vi "Serial_Init(SubVI).vi"(0 "VISA Refnum in":refnum<visa-resource-name>="COM7", 2 "wbc":dbl=1.0, 3 "delay before read (ms)":u32=265, 4 "baud rate":u32=115200, 7 "data bits":u16=8 min=5 max=8 step=1, 9 "parity":u16(ring) items=["None", "Odd", "Even", "Mark", "Space"], 11 "stop bits":u16(ring)=10 items=["1.0"=10, "1.5"=15, "2.0"=20], 12 "Success":i32, 13 "flow control":u16(ring) items=["None"=0, "XON/XOFF"=1, "RTS/CTS"=2, "DTR/DSR"=4]) -> (10 "Success_out":i32, 14 "VISA out":refnum<visa-resource-name>="COM7", 15 "read string":string, 19 "error out":errorcluster)   [LabVIEW 2017]
uses:
  <vilib>/Instr/_visa.llb/VISA Configure Serial Port (Instr).vi
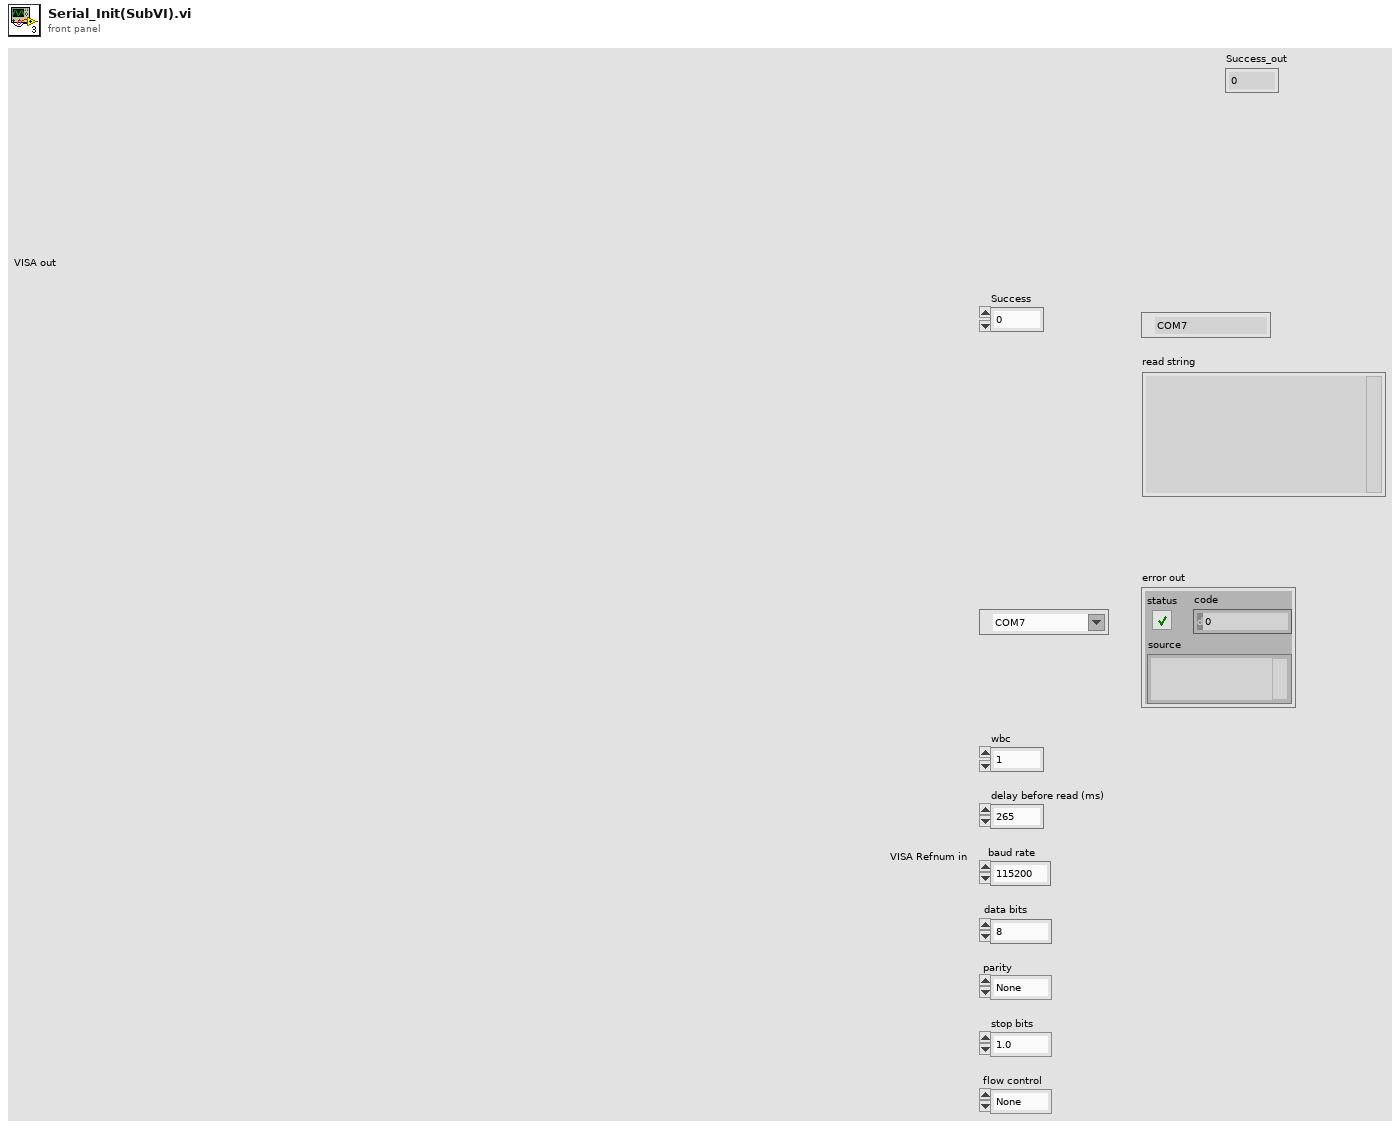
[diagram p1: front panel]
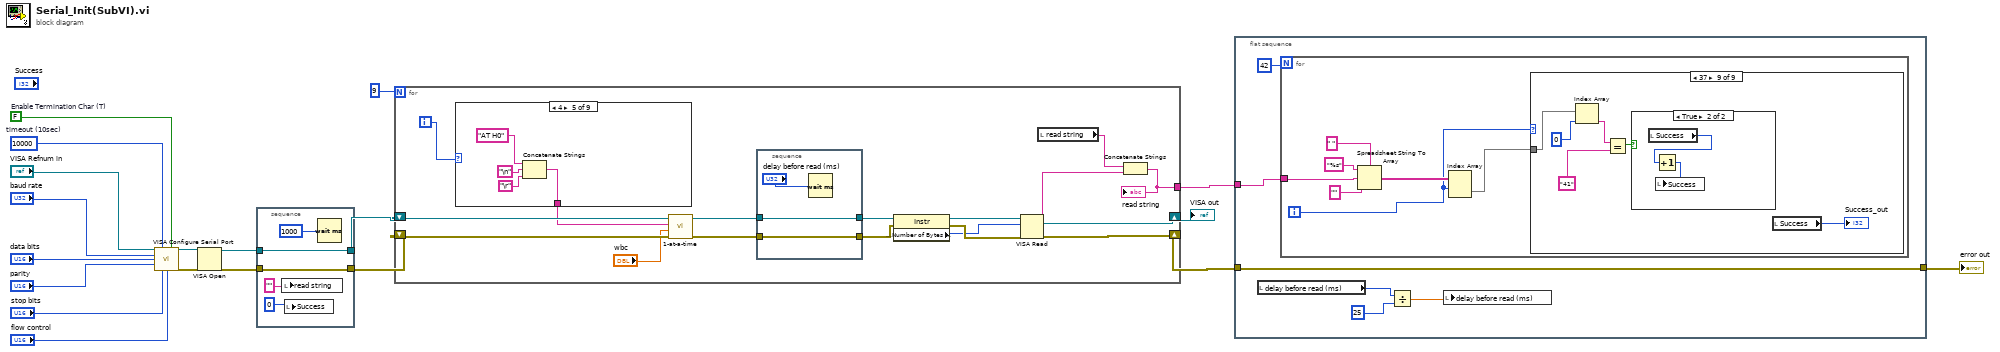
[diagram p0: block diagram]
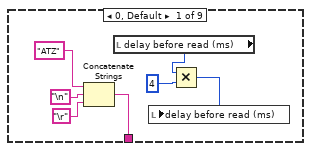
[diagram p2: hidden frame]
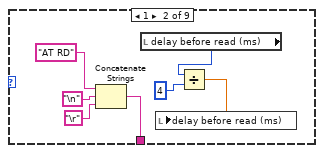
[diagram p3: hidden frame]
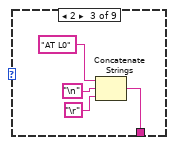
[diagram p4: hidden frame]
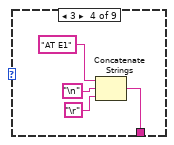
[diagram p5: hidden frame]
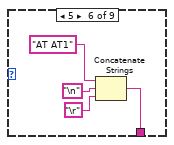
[diagram p6: hidden frame]
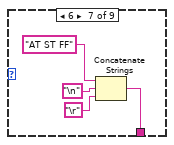
[diagram p7: hidden frame]
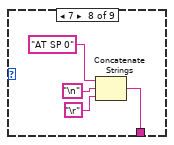
[diagram p8: hidden frame]
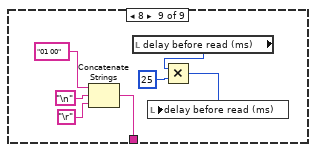
[diagram p9: hidden frame]
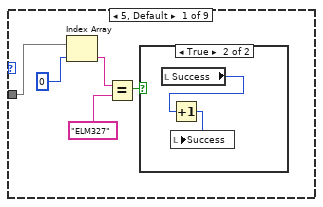
[diagram p10: hidden frame]
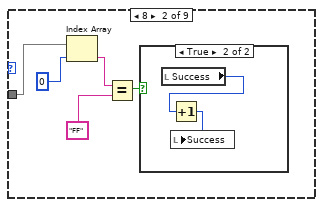
[diagram p12: hidden frame]
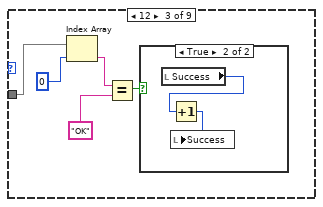
[diagram p14: hidden frame]
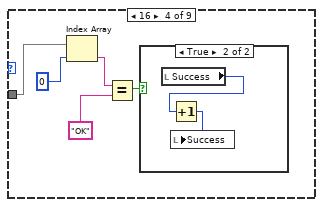
[diagram p16: hidden frame]
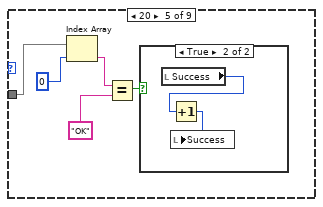
[diagram p18: hidden frame]
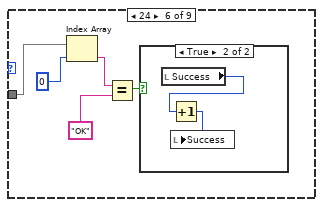
[diagram p20: hidden frame]
diagram:
  w5 = FALSE  # Enable Termination Char (T)
  w4 = u32 10000  # timeout (10sec)
  n1 = call-poly "VISA Configure Serial Port"("VISA resource name"="VISA Refnum in", "timeout (10sec)"=w4, "Enable Termination\nChar (T)"=w5, "baud rate (9600)"="baud rate", "data bits (8)"="data bits", "parity (0:none)"="parity", "stop bits (10: 1 bit)"="stop bits", "flow control (0:none)"="flow control") -> ("VISA resource name out"=w9:refnum<visa-resource-name>, "error out"=w10:errorcluster)  [unwired: 6 in]
  n2 = VISA Open(error in (no error)=w10, VISA resource name=w9) -> (VISA resource name=w11:refnum<visa-resource-name>, error out=w12:errorcluster)  [unwired: 3 in]
  n3 = stacked-sequence {
    tunnel: w12 -> [w24]
    tunnel: [w24] -> w14
    tunnel: w11 -> [w23]
    tunnel: [w23] -> w13
    frame #0 {
      n4 = local write "read string"("") -> ()
      n5 = local write "Success"(0) -> ()
      n6 = Wait (ms)(milliseconds to wait=u32 1000 ("delay before read (ms) 2")) -> ()  [unwired: 1 out]
    }
  }
  n7 = for {
    N: 9 -> [_]
    shift-right: [w29] -> w16
    shift-left: w14 -> [w40]
    shift-right: [w30] -> w15
    shift-left: w13 -> [w41]
    tunnel: [w28] -> w18
    i -> [w26]
    n8 = case shown="4" w26 {
      tunnel: [w48 w55 w59 w63 w67 w71 w75 w79 w86] -> w38
      frame 0, Default {
        n9 = Concatenate Strings("ATZ" ("string to write"), "\n", "\r") -> (w48:string)
        n10 = local read "delay before read (ms)"() -> (w43:u32)
        n11 = Multiply(x=w43, y=4) -> (x*y=w42:u32)
        n12 = local write "delay before read (ms)"(w42) -> ()
      }
      frame 1 {
        n13 = Concatenate Strings("AT RD" ("string to write"), "\n", "\r") -> (w55:string)
        n14 = local read "delay before read (ms)"() -> (w51:u32)
        n15 = Divide(x=w51, y=4) -> (x/y=w49:dbl)
        n16 = local write "delay before read (ms)"(w49) -> ()
      }
      frame 2 {
        n17 = Concatenate Strings("AT L0" ("string to write"), "\n", "\r") -> (w59:string)
      }
      frame 3 {
        n18 = Concatenate Strings("AT E1" ("string to write"), "\n", "\r") -> (w63:string)
      }
      frame 4 {
        n19 = Concatenate Strings("AT H0" ("string to write"), "\n", "\r") -> (w67:string)
      }
      frame 5 {
        n20 = Concatenate Strings("AT AT1" ("string to write"), "\n", "\r") -> (w71:string)
      }
      frame 6 {
        n21 = Concatenate Strings("AT ST FF" ("string to write"), "\n", "\r") -> (w75:string)
      }
      frame 7 {
        n22 = Concatenate Strings("AT SP 0" ("string to write"), "\n", "\r") -> (w79:string)
      }
      frame 8 {
        n23 = Concatenate Strings("01 00" ("string to write"), "\n", "\r") -> (w86:string)
        n24 = local read "delay before read (ms)"() -> (w81:u32)
        n25 = Multiply(x=w81, y=25) -> (x*y=w80:u32)
        n26 = local write "delay before read (ms)"(w80) -> ()
      }
    }
    n27 = call "1-at-a-time.vi"("error in (no error)"=w40, "Wait Between Characters(ms)"="wbc", "write buffer"=w38, "VISA resource name"=w41) -> ("error out"=w36:errorcluster, "VISA resource name out"=w37:refnum<visa-resource-name>)  [unwired: 5 in, 1 out]
    n28 = stacked-sequence {
      tunnel: w36 -> [w89]
      tunnel: [w89] -> w31
      tunnel: w37 -> [w88]
      tunnel: [w88] -> w32
      frame #0 {
        n29 = Wait (ms)(milliseconds to wait="delay before read (ms)") -> ()  [unwired: 1 out]
      }
    }
    n30 = property class="Instr"(reference=w32, error in=w31) -> (reference out=w35:refnum<visa-resource-name>, error out=w34:errorcluster, "Serial Settings:Number of Bytes at Serial Port"=w33:u32)
    n31 = VISA Read(VISA resource name=w35, byte count=w33, error in (no error)=w34) -> (VISA resource name out=w30:refnum<visa-resource-name>, read buffer=w27:string, error out=w29:errorcluster)  [unwired: 1 out]
    n32 = local read "read string"() -> (w25:string)
    n33 = Concatenate Strings(w25, w27) -> (w28:string)
    "read string" <- w28
  }
  "VISA out" <- w15
  n34 = flat-sequence {
    tunnel: w16 -> [w95]
    tunnel: [w95] -> w17
    tunnel: w18 -> [w94]
    frame #0 {
      n35 = local read "delay before read (ms)"() -> (w90:u32)
      n36 = for {
        N: 42 -> [_]
        tunnel: w94 -> [w98]
        i -> [w97]
        n37 = Spreadsheet String To Array(delimiter (Tab)=" ", format string="%s" ("spreadsheet string"), spreadsheet string=w98, array type (2D Dbl)="" ("spreadsheet string")) -> (array=w102:string[][])
        n38 = Index Array(array=w102, index (row)=w97) -> (element=w96:string[])  [unwired: 1 in]
        n39 = case shown="37" w97 {
          tunnel: w96 -> [w107 w114 w121 w128 w135 w142 w149 w156 w164]
          frame 5, Default {
            n40 = Index Array(array=w107, index=0) -> (element=w105:string)
            n41 = Equal?(x=w105, y="ELM327") -> (x = y?=w103:bool)
            n42 = case shown="True" w103 {
              frame False {
              }
              frame True {
                n43 = local read "Success"() -> (w109:i32)
                n44 = Increment(x=w109) -> (x+1=w108:i32)
                n45 = local write "Success"(w108) -> ()
              }
            }
          }
          frame 8 {
            n46 = Index Array(array=w114, index=0) -> (element=w112:string)
            n47 = Equal?(x=w112, y="FF") -> (x = y?=w110:bool)
            n48 = case shown="True" w110 {
              frame False {
              }
              frame True {
                n49 = local read "Success"() -> (w116:i32)
                n50 = Increment(x=w116) -> (x+1=w115:i32)
                n51 = local write "Success"(w115) -> ()
              }
            }
          }
          frame 12 {
            n52 = Index Array(array=w121, index=0) -> (element=w119:string)
            n53 = Equal?(x=w119, y="OK") -> (x = y?=w117:bool)
            n54 = case shown="True" w117 {
              frame False {
              }
              frame True {
                n55 = local read "Success"() -> (w123:i32)
                n56 = Increment(x=w123) -> (x+1=w122:i32)
                n57 = local write "Success"(w122) -> ()
              }
            }
          }
          frame 16 {
            n58 = Index Array(array=w128, index=0) -> (element=w126:string)
            n59 = Equal?(x=w126, y="OK") -> (x = y?=w124:bool)
            n60 = case shown="True" w124 {
              frame False {
              }
              frame True {
                n61 = local read "Success"() -> (w130:i32)
                n62 = Increment(x=w130) -> (x+1=w129:i32)
                n63 = local write "Success"(w129) -> ()
              }
            }
          }
          frame 20 {
            n64 = Index Array(array=w135, index=0) -> (element=w133:string)
            n65 = Equal?(x=w133, y="OK") -> (x = y?=w131:bool)
            n66 = case shown="True" w131 {
              frame False {
              }
              frame True {
                n67 = local read "Success"() -> (w137:i32)
                n68 = Increment(x=w137) -> (x+1=w136:i32)
                n69 = local write "Success"(w136) -> ()
              }
            }
          }
          frame 24 {
            n70 = Index Array(array=w142, index=0) -> (element=w140:string)
            n71 = Equal?(x=w140, y="OK") -> (x = y?=w138:bool)
            n72 = case shown="True" w138 {
              frame False {
              }
              frame True {
                n73 = local read "Success"() -> (w144:i32)
                n74 = Increment(x=w144) -> (x+1=w143:i32)
                n75 = local write "Success"(w143) -> ()
              }
            }
          }
          frame 28 {
            n76 = Index Array(array=w149, index=0) -> (element=w147:string)
            n77 = Equal?(x=w147, y="OK") -> (x = y?=w145:bool)
            n78 = case shown="True" w145 {
              frame False {
              }
              frame True {
                n79 = local read "Success"() -> (w151:i32)
                n80 = Increment(x=w151) -> (x+1=w150:i32)
                n81 = local write "Success"(w150) -> ()
              }
            }
          }
          frame 36 {
            n82 = Index Array(array=w156, index=0) -> (element=w154:string)
            n83 = Equal?(x=w154, y="SEARCHING...") -> (x = y?=w152:bool)
            n84 = case shown="True" w152 {
              frame False {
              }
              frame True {
                n85 = local read "Success"() -> (w158:i32)
                n86 = Increment(x=w158) -> (x+1=w157:i32)
                n87 = local write "Success"(w157) -> ()
              }
            }
          }
          frame 37 {
            n88 = Index Array(array=w164, index=0) -> (element=w162:string)
            n89 = Equal?(x=w162, y="41") -> (x = y?=w160:bool)
            n90 = case shown="True" w160 {
              frame False {
              }
              frame True {
                n91 = local read "Success"() -> (w166:i32)
                n92 = Increment(x=w166) -> (x+1=w165:i32)
                n93 = local write "Success"(w165) -> ()
              }
            }
            n94 = local read "Success"() -> (→"Success_out":i32)
          }
        }
      }
      n95 = Divide(x=w90, y=25) -> (x/y=w91:dbl)
      n96 = local write "delay before read (ms)"(w91) -> ()
    }
  }
  "error out" <- w17
